vi "queue_array_front.vi"(8 "error in":errorcluster, 10 "array":string[](array[string])=["Data: Initialize", "Initialize Core Data", "Data: Get Case Strings", "Data: Get Case Documentation", "UI: Initialize", "UI: Front Panel State >> Open", "Delay >> 1000"], 11 "queue in":refnum<queue>) -> (0 "error out":errorcluster, 3 "queue out":refnum<queue>)   [LabVIEW 2012]
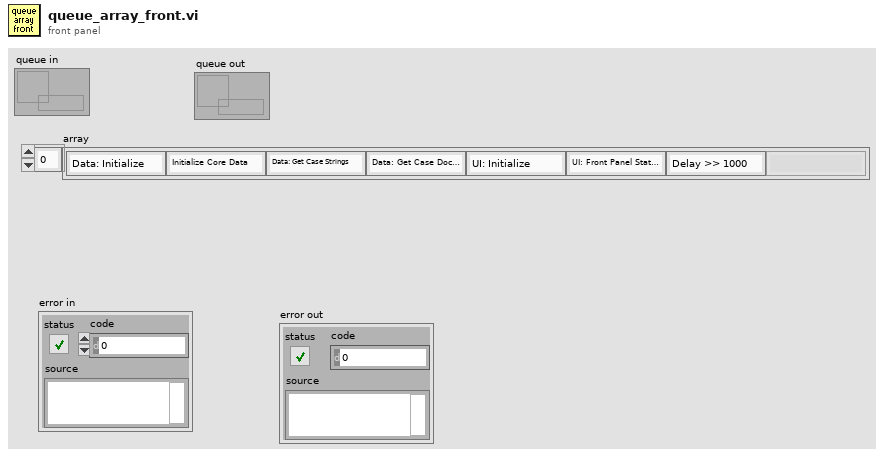
[diagram p1: front panel]
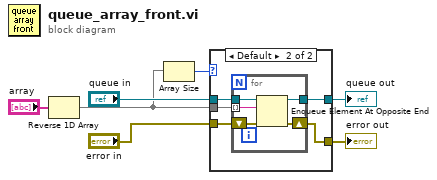
[diagram p0: block diagram]
diagram:
  n1 = Reverse 1D Array(array="array") -> (reversed array=w2:string[])
  n2 = Array Size(array=w2) -> (size(s)=w1:i32)
  n3 = case shown="Default" w1 {
    tunnel: w2 -> [_ w14]
    tunnel: [w9 w13] -> w7
    tunnel: [w8 w12] -> w6
    tunnel: "queue in" -> [w9 w11]
    tunnel: "error in" -> [w8 w10]
    frame 0 {
    }
    frame Default {
      n4 = for {
        tunnel: [w19] -> w13
        tunnel: w11 -> [w18]
        shift-right: [w16] -> w12
        shift-left: w10 -> [w17]
        tunnel: w14 -> [w15] mode=indexing
        n5 = Enqueue Element At Opposite End(queue=w18, element=w15, error in (no error)=w17) -> (queue out=w19:refnum<queue>, error out=w16:errorcluster)  [unwired: 1 in, 1 out]
      }
    }
  }
  "queue out" <- w7
  "error out" <- w6
